vi "CC Script to Tree.vi"(7 "Calling Script":string, 8 "error in (no error)":errorcluster, 9 "Row":i32, 10 "Tree ref":refnum<vi>, 11 "Script":T1) -> (0 "error out":errorcluster, 3 "table":string[][](array[string]))   [LabVIEW 2020]
uses:
  typedefs/CC cluster Script.ctl
  typedefs/CC Script Step.ctl
  typedefs/CC enum Script Action.ctl
  typedefs/CC cluster Object.ctl
  typedefs/CCenum Object Type.ctl
  typedefs/CCenum Object Position Type.ctl
  typedefs/CC cluster sidereal rate.ctl
  typedefs/CC cluster RA and DEC.ctl
  typedefs/cc cluster muRA muDEC.ctl
  typedefs/CC cluster tplane.ctl
  typedefs/CC cluster Exposure.ctl
  typedefs/CC Dithering.ctl
  typedefs/CC cluster Offset Dithering.ctl
  typedefs/CC Dithering Offsets.ctl
  typedefs/CC cluster Acquire Parameters.ctl
  typedefs/CC cluster Filter Wheel Parameters.ctl
  Focus/Focus cluster MoveFocus Command Parameters.ctl
  typedefs/CC cluster Pause Parameters.ctl
panel:
  in  "Tree":string(tree)
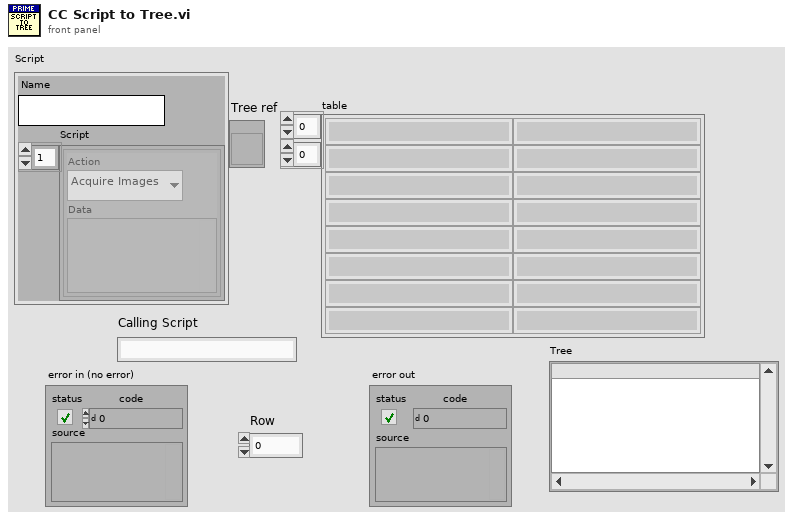
[diagram p1: front panel]
types:
  T1 = typedef "CC cluster Script.ctl" = cluster{"Name":string, "Script":T2[]}
  T2 = typedef "CC Script Step.ctl" = cluster{"Action":T3, "Data":variant}
  T3 = typedef "CC enum Script Action.ctl" = enum16{"Noop", "Define Object", "Define Exposure", "Define Dithering", "Acquire Images", "Set Filter Wheel", "Telescope Home", "Telescope Move", "Focus Move Relative", "Focus Move Absolute", "Focus Set Home", "Macro", "Pause", "Ask User", "Define Random Dither"}
  T4 = typedef "CC cluster Object.ctl" = cluster{"Object":cluster{"Name":string, "Type":T5, "Position Type":T6}, "Sidereal Rate":T7, "RA and DEC":T8, "muRA muDEC Epoch":T9, "tplane offsets":T10}
  T5 = typedef "CCenum Object Type.ctl" = enum16{"Standard", "Science"}
  T6 = typedef "CCenum Object Position Type.ctl" = enum16{"RA-DEC", "muRA-muDEC-epoch"}
  T7 = typedef "CC cluster sidereal rate.ctl" = cluster{"dRA":dbl, "dDEC":dbl}
  T8 = typedef "CC cluster RA and DEC.ctl" = cluster{"RA":dbl, "DEC":dbl}
  T9 = typedef "cc cluster muRA muDEC.ctl" = cluster{"muRA":dbl, "muDEC":dbl, "Epoch":dbl}
  T10 = typedef "CC cluster tplane.ctl" = cluster{"xi":dbl, "eta":dbl}
  T11 = typedef "CC cluster Exposure.ctl" = cluster{"Number":i32, "Readout Groups":i32, "Readouts per Group":i32, "Time Between Groups":dbl, "Time Between Readouts":dbl, "Name":string}
  T12 = typedef "CC Dithering.ctl" = cluster{"Name":string, "Dithering Offsets":T13}
  T13 = typedef "CC cluster Offset Dithering.ctl" = cluster{"Offsets":T14[]}
  T14 = typedef "CC Dithering Offsets.ctl" = cluster{"DEC":dbl, "RA":dbl}
  T15 = typedef "CC cluster Acquire Parameters.ctl" = cluster{"Object":string, "Exposure":string, "Dithering":string}
  T16 = typedef "CC cluster Filter Wheel Parameters.ctl" = cluster{"Wheel":i32, "Filter":i32}
  T17 = typedef "Focus cluster MoveFocus Command Parameters.ctl" = cluster{"Motor":i32, "Position":i32}
  T18 = typedef "CC cluster Pause Parameters.ctl" = cluster{"Time (s)":dbl}
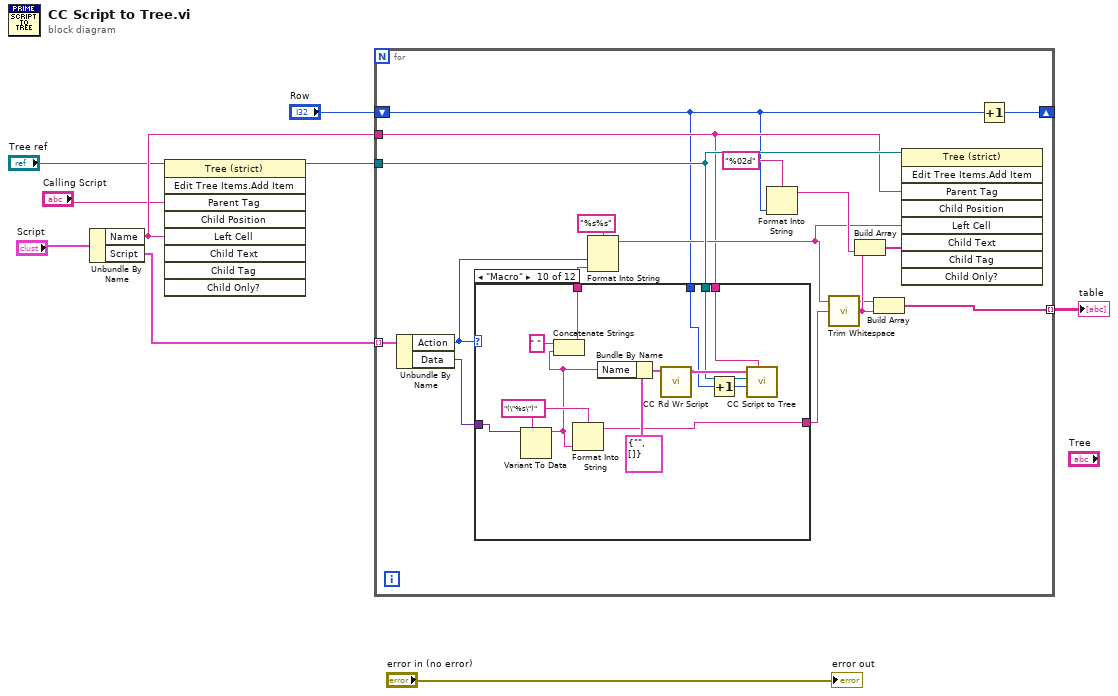
[diagram p0: block diagram]
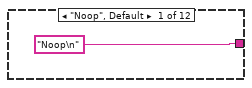
[diagram p2: hidden frame]
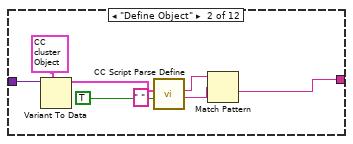
[diagram p3: hidden frame]
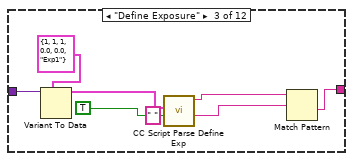
[diagram p4: hidden frame]
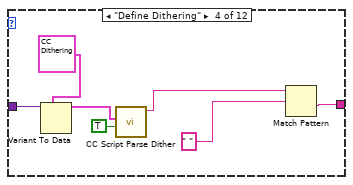
[diagram p5: hidden frame]
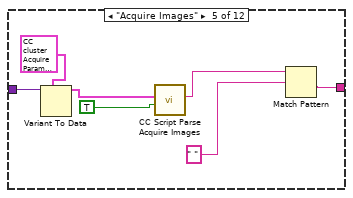
[diagram p6: hidden frame]
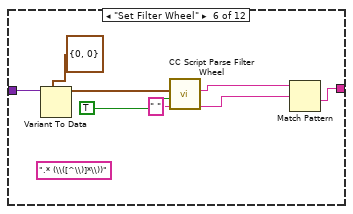
[diagram p7: hidden frame]
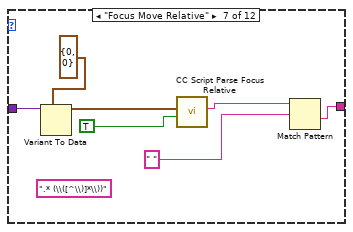
[diagram p8: hidden frame]
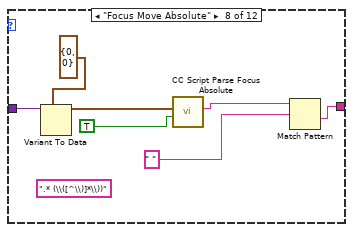
[diagram p9: hidden frame]
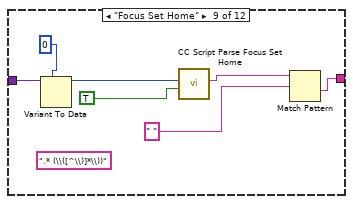
[diagram p10: hidden frame]
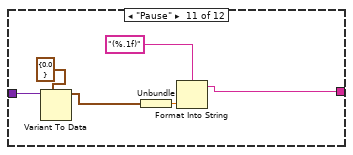
[diagram p11: hidden frame]
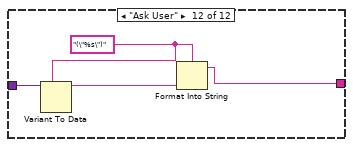
[diagram p12: hidden frame]
diagram:
  n1 = Unbundle By Name("Script") -> ("Name"=w7:string, "Script"=w5:T2[])
  n2 = invoke on="Invoke Node" class="Tree (strict)" method="Edit Tree Items.Add Item"(reference="Tree ref", "Parent Tag"="Calling Script", "Left Cell"=w7) -> (reference out=w3:refnum<vi>)  [unwired: 6 in, 8 out]
  n3 = for {
    tunnel: w5 -> [w25] mode=indexing
    tunnel: [w18] -> w8 mode=indexing
    tunnel: w7 -> [w12]
    tunnel: w3 -> [w17]
    shift-right: [w10] -> _
    shift-left: "Row" -> [w11]
    n4 = Unbundle By Name(w25) -> ("Action"=w22:T3, "Data"=w23:variant)
    n5 = case shown="\"Macro\"" w22 {
      tunnel: w23 -> [_ w33 w40 w47 w54 w61 w68 w75 w82 w94 w101 w105]
      tunnel: ["Noop\n" ("string") w28 w34 w41 w48 w55 w66 w73 w80 w92 w96 w102] -> w21
      tunnel: w17 -> [_ _ _ _ _ _ _ _ _ w89 _ _]
      tunnel: w11 -> [_ _ _ _ _ _ _ _ _ w88 _ _]
      tunnel: [_ _ _ _ _ _ _ _ _ w84 _ _] -> w14
      tunnel: w12 -> [_ _ _ _ _ _ _ _ _ w83 _ _]
      frame "Noop", Default {
      }
      frame "Define Object" {
        n6 = Variant To Data(type=T4 {"Object"={"Name"="", "Type"=enum."Standard", "Position Type"=enum."RA-DEC"}, "Sidereal Rate"={"dRA"=0.0, "dDEC"=0.0}, "RA and DEC"={"RA"=0.0, "DEC"=0.0}, "muRA muDEC Epoch"={"muRA"=0.0, "muDEC"=0.0, "Epoch"=0.0}, "tplane offsets"={"xi"=0.0, "eta"=0.0}} ("Object"), Variant=w33) -> (data=w31:T4)  [unwired: 1 in, 1 out]
        n7 = call "CC Script Parse Define.vi"("To String?"=TRUE, "Object in"=w31) -> ("Script"=w29:string)  [unwired: 6 in, 3 out]
        n8 = Match Pattern(string=w29, regular expression=" ") -> (after substring=w28:string)  [unwired: 1 in, 3 out]
      }
      frame "Define Exposure" {
        n9 = Variant To Data(type=T11 {"Number"=1, "Readout Groups"=1, "Readouts per Group"=1, "Time Between Groups"=0.0, "Time Between Readouts"=0.0, "Name"="Exp1"} ("Exposure in"), Variant=w40) -> (data=w38:T11)  [unwired: 1 in, 1 out]
        n10 = call "CC Script Parse Define Exp.vi"("To String?"=TRUE, "Exposure in"=w38) -> ("Script String out"=w35:string)  [unwired: 6 in, 3 out]
        n11 = Match Pattern(string=w35, regular expression=" ") -> (after substring=w34:string)  [unwired: 1 in, 3 out]
      }
      frame "Define Dithering" {
        n12 = Variant To Data(type=T12 {"Name"="", "Dithering Offsets"={"Offsets"=[{"DEC"=0.0, "RA"=0.0}, {"DEC"=-10.0, "RA"=-10.0}]}} ("Dithering Offsets in"), Variant=w47) -> (data=w45:T12)  [unwired: 1 in, 1 out]
        n13 = call "CC Script Parse Dither.vi"("To String?"=TRUE, "Dithering in"=w45) -> ("resulting string"=w42:string)  [unwired: 7 in, 2 out]
        n14 = Match Pattern(string=w42, regular expression=" ") -> (after substring=w41:string)  [unwired: 1 in, 3 out]
      }
      frame "Acquire Images" {
        n15 = Variant To Data(type=T15 {"Object"="Alpha1234", "Exposure"="Exp1", "Dithering"="Dither2"} ("Acquire Parameters in"), Variant=w54) -> (data=w52:T15)  [unwired: 1 in, 1 out]
        n16 = call "CC Script Parse Acquire Images.vi"("To Script?"=TRUE ("To String?"), "Acquire Parameters in"=w52) -> ("Script out"=w49:string)  [unwired: 7 in, 2 out]
        n17 = Match Pattern(string=w49, regular expression=" ") -> (after substring=w48:string)  [unwired: 1 in, 3 out]
      }
      frame "Set Filter Wheel" {
        (unwired) ".* (\\([^\\)]*\\))" ("regular expression")
        n18 = Variant To Data(type=T16 {"Wheel"=0, "Filter"=0} ("Acquire Parameters in"), Variant=w61) -> (data=w59:T16)  [unwired: 1 in, 1 out]
        n19 = call "CC Script Parse Filter Wheel.vi"("To Script?"=TRUE ("To String?"), "Filter Wheel parameters in"=w59) -> ("Script Out"=w56:string)  [unwired: 7 in, 2 out]
        n20 = Match Pattern(string=w56, regular expression=" ") -> (after substring=w55:string)  [unwired: 1 in, 3 out]
      }
      frame "Focus Move Relative" {
        (unwired) ".* (\\([^\\)]*\\))" ("regular expression")
        n21 = Variant To Data(type=T17 {"Motor"=0, "Position"=0} ("Cluster"), Variant=w68) -> (data=w64:T17)  [unwired: 1 in, 1 out]
        n22 = call "CC Script Parse Focus Relative.vi"("To Script?"=TRUE ("To String?"), "Move parm in"=w64) -> ("Script Out"=w62:string)  [unwired: 7 in, 2 out]
        n23 = Match Pattern(string=w62, regular expression=" ") -> (after substring=w66:string)  [unwired: 1 in, 3 out]
      }
      frame "Focus Move Absolute" {
        (unwired) ".* (\\([^\\)]*\\))" ("regular expression")
        n24 = Variant To Data(type=T17 {"Motor"=0, "Position"=0} ("Cluster"), Variant=w75) -> (data=w71:T17)  [unwired: 1 in, 1 out]
        n25 = call "CC Script Parse Focus Absolute.vi"("To Script?"=TRUE ("To String?"), "Move parm in"=w71) -> ("Script Out"=w69:string)  [unwired: 7 in, 2 out]
        n26 = Match Pattern(string=w69, regular expression=" ") -> (after substring=w73:string)  [unwired: 1 in, 3 out]
      }
      frame "Focus Set Home" {
        (unwired) ".* (\\([^\\)]*\\))" ("regular expression")
        n27 = Variant To Data(type=0 ("Motor"), Variant=w82) -> (data=w78:i32)  [unwired: 1 in, 1 out]
        n28 = call "CC Script Parse Focus Set Home.vi"("To Script?"=TRUE ("To String?"), "Set Home parm in"=w78) -> ("Script Out"=w76:string)  [unwired: 7 in, 2 out]
        n29 = Match Pattern(string=w76, regular expression=" ") -> (after substring=w80:string)  [unwired: 1 in, 3 out]
      }
      frame "Macro" {
        w95 = "(\"%s\")" ("format string")
        n30 = Variant To Data(type=w95, Variant=w94) -> (data=w85:string)  [unwired: 1 in, 1 out]
        n31 = Concatenate Strings(" " ("string"), w85) -> (w84:string)
        n32 = Format Into String(format string=w95, w85) -> (resulting string=w92:string)  [unwired: 2 in, 1 out]
        n33 = Bundle By Name(cluster=T1 {"Name"="", "Script"=[]} ("Script"), "Name"=w85) -> (w91:T1)
        n34 = call "CC Rd Wr Script.vi"("Script"=w91) -> ("Script"=w90:T1)  [unwired: 6 in, 4 out]
        n35 = Increment(x=w88) -> (x+1=w87:i32)
        n36 = call "CC Script to Tree.vi"("Calling Script"=w83, "Row"=w87, "Tree ref"=w89, "Script"=w90) -> ()  [unwired: 6 in, 2 out]
      }
      frame "Pause" {
        n37 = Variant To Data(type=T18 {"Time (s)"=0.0} ("Acquire Parameters in"), Variant=w101) -> (data=w98:T18)  [unwired: 1 in, 1 out]
        n38 = Unbundle(w98) -> ("Time (s)"=w97:dbl)
        n39 = Format Into String(format string="(%.1f)", w97) -> (resulting string=w96:string)  [unwired: 2 in, 1 out]
      }
      frame "Ask User" {
        w104 = "(\"%s\")" ("format string")
        n40 = Variant To Data(type=w104, Variant=w105) -> (data=w103:string)  [unwired: 1 in, 1 out]
        n41 = Format Into String(format string=w104, w103) -> (resulting string=w102:string)  [unwired: 2 in, 1 out]
      }
    }
    n42 = Format Into String(format string="%s%s", w22, w14) -> (resulting string=w13:string)  [unwired: 2 in, 1 out]
    n43 = Format Into String(format string="%02d", w11) -> (resulting string=w16:string)  [unwired: 2 in, 1 out]
    n44 = call <vilib>:"Trim Whitespace.vi"("string"=w21) -> ("trimmed string"=w20:string)  [unwired: 1 in]
    n45 = Build Array(w20, w16) -> (w19:string[])
    n46 = Build Array(w13, w20) -> (w18:string[])
    n47 = invoke on="Invoke Node" class="Tree (strict)" method="Edit Tree Items.Add Item"(reference=w17, "Parent Tag"=w12, "Left Cell"=w13, "Child Text"=w19) -> ()  [unwired: 5 in, 9 out]
    n48 = Increment(x=w11) -> (x+1=w10:i32)
  }
  "table" <- w8
  "error out" <- "error in (no error)"
